vi "Setup subWorkers.vi"(8 "error in":errorcluster, 11 "ChartView Worker in":refnum<class "ChartView Worker.lvclass">) -> (0 "error out":errorcluster, 3 "ChartView Worker out":refnum<class "ChartView Worker.lvclass">)   [LabVIEW 2018, in "ChartView Worker.lvclass"]
doc: "<b>Note: Do not change the code in this VI!</b>\nThis VI performs a setup of all the statically-linked subWorkers that belong to the Worker that calls this VI. This VI is created automatically by the 'Create/Add Worker' tool and must be called <b>before</b> any statically linked subWorkers are called."
uses:
  ChartView Worker.lvclass
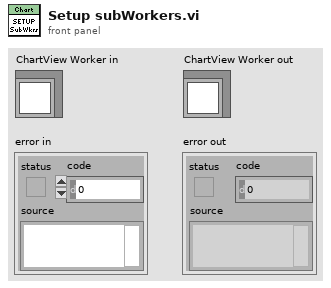
[diagram p1: front panel]
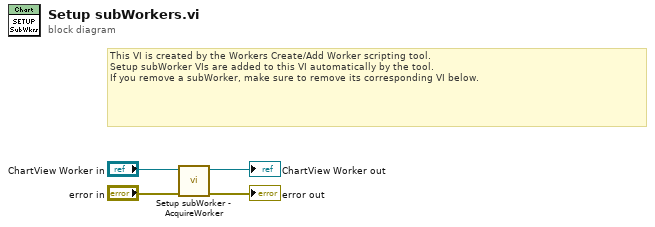
[diagram p0: block diagram]
diagram:
  # "This VI is created by the Workers Create/Add Worker scripting tool.\nSetup subWorker VIs are added to this VI automatically by the tool.\nIf you remove a subWorker, make sure to remove its corresponding VI below."
  n1 = call "Setup subWorker - AcquireWorker.vi"("error in"="error in", "ChartView Worker in"="ChartView Worker in") -> ("error out"=→"error out":errorcluster, "ChartView Worker out"=→"ChartView Worker out":refnum<class "ChartView Worker.lvclass">)  [unwired: 8 in]
